vi "Write currentTimeActivity.vi"(8 "error in (no error)":errorcluster, 10 "ActivityValues":T1, 11 "TCSIersStatus in":refnum<class "TCSIersStatus.lvclass">) -> (0 "error out":errorcluster, 3 "TCSIersStatus out":refnum<class "TCSIersStatus.lvclass">)   [LabVIEW 2014, in "TCSDataDefinitions.lvlib" / "TCSTimeComponentStatus.lvlib" / "TCSIersStatus.lvclass"]
uses:
  TCSIersStatus.lvclass
  Enumerations/ActivityValues.ctl
  TCSIersStatus.lvclass/TCSIersStatus.ctl
  TCSTimeComponentStatus.lvlib
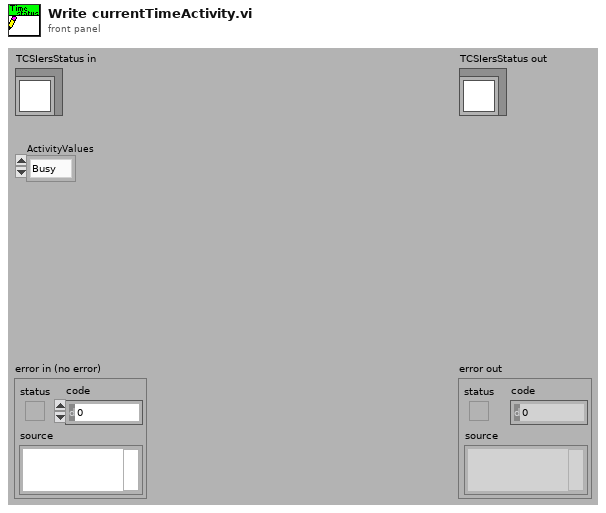
[diagram p1: front panel]
types:
  T1 = typedef "TCSDataDefinitions.lvlib/TCSTimeComponentStatus.lvlib/ActivityValues.ctl" = enum16{"Busy", "Error", "Idle"}
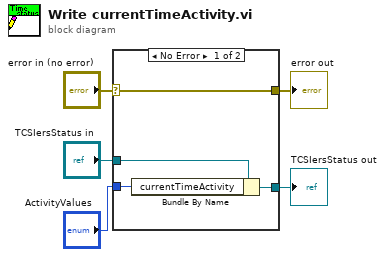
[diagram p0: block diagram]
diagram:
  n1 = case shown="No Error" "error in (no error)" {
    selector: "error in (no error)" -> [w9 w10]
    tunnel: [w9 w10] -> w4
    tunnel: [w7 w11] -> w2
    tunnel: "TCSIersStatus in" -> [w8 w11]
    tunnel: "ActivityValues" -> [w6 _]
    frame No Error {
      n2 = Bundle By Name(cluster=w8, "currentTimeActivity"=w6) -> (w7:refnum<class "TCSIersStatus.lvclass">)
    }
    frame Error {
    }
  }
  "error out" <- w4
  "TCSIersStatus out" <- w2
